vi "Python String to LabVIEW Data (VEnum).vi"(8 "error in (no error)":errorcluster, 9 "type (VEnum)":variant, 10 "Python String":string) -> (0 "error out":errorcluster, 2 "LabVIEW Data":variant)   [LabVIEW 2020, in "jki_python_data_tools.lvlib"]
doc: "Reads a value associated with key in a specified section of the configuration data identified by refnum. If \"key\" input is not specified, the name of the variant object is used as the key. the \"found?\" output will be TRUE for compount objects (clusters) only if all elements (recursively) are found.\n\nFor example a Boolean named \"Enable\" with a value of TRUE would correspond to the key-value pair:\n\nEnable=TRUE"
uses:
  jki_python_data_tools.lvlib
  <userlib>/_OpenG.lib/lvdata/lvdata.llb/openg_variant.lvlib
panel:
  # "Copyright © 2003-2009 JKI. All rights reserved.\n\nAuthor:\nPhilippe Guerit [philippe.guerit@jameskring.com]\nJim Kring [jim.kring@jameskring.com]\n\nThis library is provided \"AS IS\" ,WITHOUT WARRANTIES OR \nCONDITIONS OF ANY KIND, either express or implied.\n\nJames Kring, Inc. -- http://www.jameskring.com"
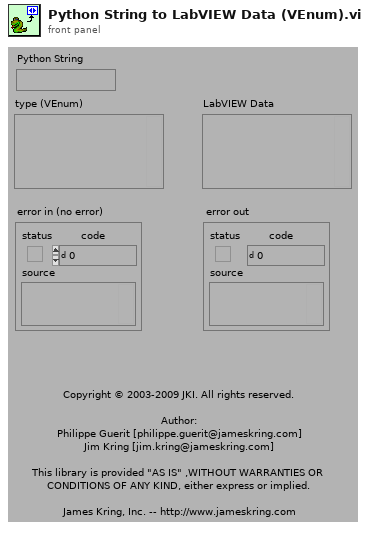
[diagram p1: front panel]
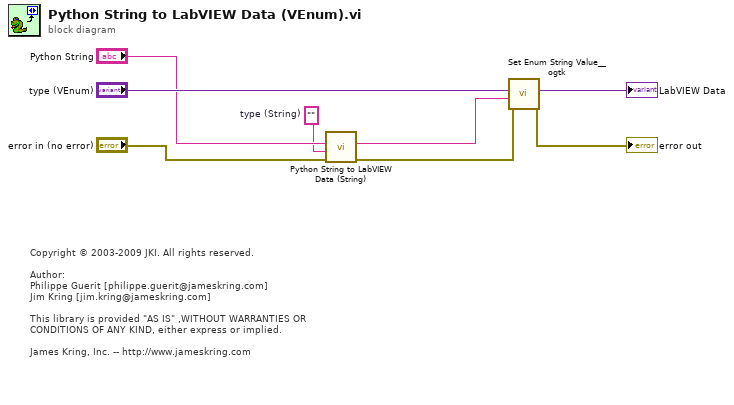
[diagram p0: block diagram]
diagram:
  w1 = ""  # type (String)
  # "Copyright © 2003-2009 JKI. All rights reserved.\n\nAuthor:\nPhilippe Guerit [philippe.guerit@jameskring.com]\nJim Kring [jim.kring@jameskring.com]\n\nThis library is provided \"AS IS\" ,WITHOUT WARRANTIES OR \nCONDITIONS OF ANY KIND, either express or implied.\n\nJames Kring, Inc. -- http://www.jameskring.com"
  n1 = call "Python String to LabVIEW Data (String).vi"("error in (no error)"="error in (no error)", "type (String)"=w1, "Python String"="Python String") -> ("error out"=w5:errorcluster, "LabVIEW Data"=w2:string)  [unwired: 7 in]
  n2 = call <userlib>:"Set Enum String Value__ogtk.vi"("error in (no error)"=w5, "String Value"=w2, "Default Enum Value"="type (VEnum)") -> ("error out"=→"error out":errorcluster, "Enum"=→"LabVIEW Data":variant)  [unwired: 7 in]
